vi "action.vi"(0 "HGF_SVVisitor_deregister in":refnum<class "HGF_SVMonitorVisitor_deregister.lvclass">, 2 "HGF_Visitable":refnum<class "HGF_Visitable.lvclass">, 5 "error in (no error)":errorcluster) -> (14 "HGF_SVVisitor_deregister out":refnum<class "HGF_SVMonitorVisitor_deregister.lvclass">, 16 "dup HGF_Visitable":refnum<class "HGF_Visitable.lvclass">, 19 "error out":errorcluster)   [LabVIEW 2012, in "HGF_SV.lvlib" / "HGF_SVMonitorVisitor_deregister.lvclass"]
doc: "This is a dynamic dispatch VI that is called from Visitor.visit(). It will call member VIs of Visitable to perform the requested action which means: calling public methods of Visitable child class.\n\n<B>Hint:</B> This method is abstract and need to be implemented by child classes."
uses:
  HGF_SVMonitorVisitor_deregister.lvclass
  HGF_BaseClasses/HGF_Visitable/HGF_Visitable.lvclass
  HGF_Monitor/HGF_Monitor.lvclass
  HGF_SVMonitorVisitor/HGF_SVMonitorVisitor.lvclass
  HGF_SVMonitorVisitor_deregister.lvclass/HGF_SVMonitorVisitor_deregister.ctl
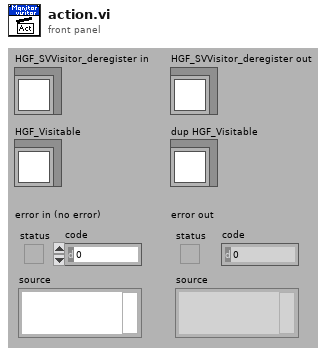
[diagram p1: front panel]
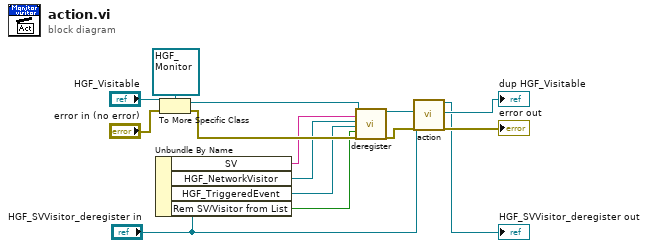
[diagram p0: block diagram]
diagram:
  n1 = Unbundle By Name("HGF_SVVisitor_deregister in") -> ("SV"=w2:string, "HGF_NetworkVisitor"=w3:refnum<class "HGF_NetworkVisitor.lvclass">, "HGF_TriggeredEvent"=w4:refnum<class "HGF_TriggeredEvent.lvclass">, "Rem SV/Visitor from List"=w5:bool)
  n2 = To More Specific Class(target class=refnum<class "HGF_Monitor.lvclass"> refnum ("HGF_SV.lvlib:HGF_Monitor.lvclass"), reference="HGF_Visitable", error in="error in (no error)") -> (specific class reference=w10:refnum<class "HGF_Monitor.lvclass">, error out=w6:errorcluster)
  n3 = call-dynamic "deregister.vi"("HGF_Monitor in"=w10, "Variable"=w2, "HGF_NetworkVisitor"=w3, "HGF_TriggeredEvent"=w4, "Rem SV/Visitor from List"=w5, "error in (no error)"=w6) -> ("HGF_Monitor out"=w8:refnum<class "HGF_Monitor.lvclass">, "error out"=w7:errorcluster)  [unwired: 12 in]
  n4 = call-parent "action.vi"("HGF_SVVisitor_runMon in"="HGF_SVVisitor_deregister in", "HGF_Visitable"=w8, "error in (no error)"=w7) -> ("HGF_SVVisitor_runMon out"=→"HGF_SVVisitor_deregister out":refnum<class "HGF_SVMonitorVisitor_deregister.lvclass">, "dup HGF_Visitable"=→"dup HGF_Visitable":refnum<class "HGF_Visitable.lvclass">, "error out"=→"error out":errorcluster)  [unwired: 14 in]
